vi "Autobalance State 2 Cal Autobalance State.vi"(10 "Autobalance State In":T1[](array[typedef])) -> (2 "Cal Autobalance State":T5)   [LabVIEW 2009]
uses:
  Cal Autobalance State.ctl
  Apps/Yes No Button.ctl
  Autobalance/Autobalance Stage.ctl
  Autobalance/Autobalance Status Data.ctl
  Autobalance/Autobalance Data Point.ctl
panel:
  # "Cmd"
  # "Servo"
  # "Cmd"
  # "Servo"
  # "Is Balanced"
  # "State"
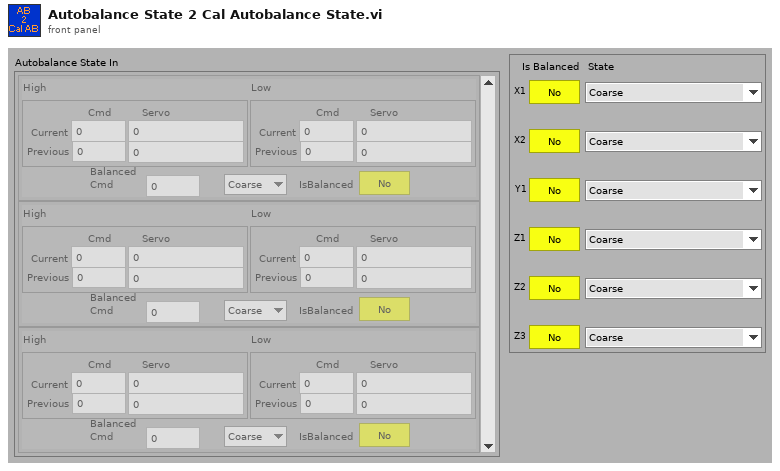
[diagram p1: front panel]
types:
  T1 = typedef "Autobalance Status Data.ctl" = cluster{"IsBalanced":T2, "Autobalance Stage":T3, "High":T4, "Low":T4, "Balanced \nCmd":dbl}
  T2 = typedef "Yes No Button.ctl" = bool
  T3 = typedef "Autobalance Stage.ctl" = enum16{"Coarse", "Fine", "Backing Up", "Done"}
  T4 = typedef "Autobalance Data Point.ctl" = cluster{"cCmd":dbl, "cServo":dbl, "pCmd":dbl, "pServo":dbl}
  T5 = typedef "Cal Autobalance State.ctl" = cluster{"X1 IsBalanced":T2, "X1 State":T3, "X2 IsBalanced":T2, "X2 State":T3, "Y1 IsBalanced":T2, "Y1 State":T3, "Z1 IsBalanced":T2, "Z1 State":T3, "Z2 IsBalanced":T2, "Z2 State":T3, "Z3 IsBalanced":T2, "Z3 State":T3}
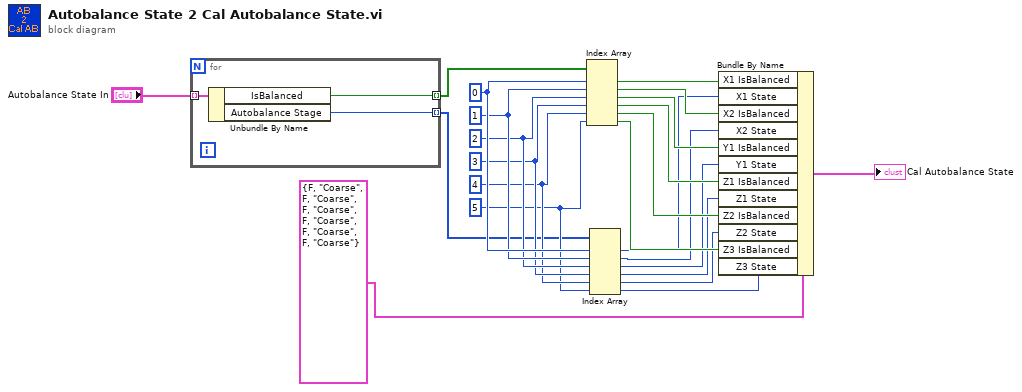
[diagram p0: block diagram]
diagram:
  w15 = 5 ("index")
  w16 = 4 ("index")
  w17 = 3 ("index")
  w18 = 2 ("index")
  w19 = 1 ("index")
  w20 = 0 ("index")
  n1 = for {
    tunnel: "Autobalance State In" -> [w26] mode=indexing
    tunnel: [w25] -> w22 mode=indexing
    tunnel: [w24] -> w14 mode=indexing
    n2 = Unbundle By Name(w26) -> ("IsBalanced"=w25:T2, "Autobalance Stage"=w24:T3)
  }
  n3 = Index Array(array=w22, index #1=w20, index #2=w19, index #3=w18, index #4=w17, index #5=w16, index #6=w15) -> (element #1=w13:T2, element #2=w12:T2, element #3=w11:T2, element #4=w10:T2, element #5=w9:T2, element #6=w8:T2)
  n4 = Index Array(array=w14, index #1=w20, index #2=w19, index #3=w18, index #4=w17, index #5=w16, index #6=w15) -> (element #1=w7:T3, element #2=w6:T3, element #3=w5:T3, element #4=w4:T3, element #5=w3:T3, element #6=w2:T3)
  n5 = Bundle By Name(cluster=T5 {"X1 IsBalanced"=FALSE, "X1 State"=enum."Coarse", "X2 IsBalanced"=FALSE, "X2 State"=enum."Coarse", "Y1 IsBalanced"=FALSE, "Y1 State"=enum."Coarse", "Z1 IsBalanced"=FALSE, "Z1 State"=enum."Coarse", "Z2 IsBalanced"=FALSE, "Z2 State"=enum."Coarse", "Z3 IsBalanced"=FALSE, "Z3 State"=enum."Coarse"} ("Cal Autobalance State"), "X1 IsBalanced"=w13, "X1 State"=w7, "X2 IsBalanced"=w12, "X2 State"=w6, "Y1 IsBalanced"=w11, "Y1 State"=w5, "Z1 IsBalanced"=w10, "Z1 State"=w4, "Z2 IsBalanced"=w9, "Z2 State"=w3, "Z3 IsBalanced"=w8, "Z3 State"=w2) -> (→"Cal Autobalance State":T5)
